vi "interface_configuration.vi"(8 "error in (no error)":errorcluster, 11 "config in":T1) -> (0 "error out":errorcluster, 3 "config out":T1)   [LabVIEW 2015, in "lv-builder-default.lvlib"]
uses:
  lv-builder-default.lvlib
  public/_controls/post_action_lvlib.ctl
  public/_controls/post_action_installer.ctl
  public/_controls/post_action_application.ctl
  public/_controls/post_action_zip.ctl
  public/_controls/configuration.ctl
  <vilib>/Utility/error.llb/Error Cluster From Error Code.vi
  <vilib>/ErrorRing/Error Ring.xnode
panel:
  in  "version":string caption="Version"
  in  "distribution_folder":path caption="Distribution Folder"
  in  "dependencies_folder":path caption="Dependencies Folder"
  in  "bin_folder":path caption="Bin Path"
  in  "application_post_action":T2 caption="Application Post Action"
  in  "cancel":bool
  in  "save":bool
  in  "installer_post_file":path caption="Installer Post File"
  in  "zip_move_directory":path caption="Archive Directory"
  in  "zip_post_action":T3 caption="Archive Post Action"
  in  "installer_post_action":T4 caption="Installer Post Action"
  in  "update_version_vi":path caption="Update Version VI"
  in  "lvlibp_move_directory":path caption="lvlibp Directory"
  in  "lvlib_move_directory":path caption="lvlib Directory"
  in  "lvlib_post_action":T5 caption="LVLIB Post Action"
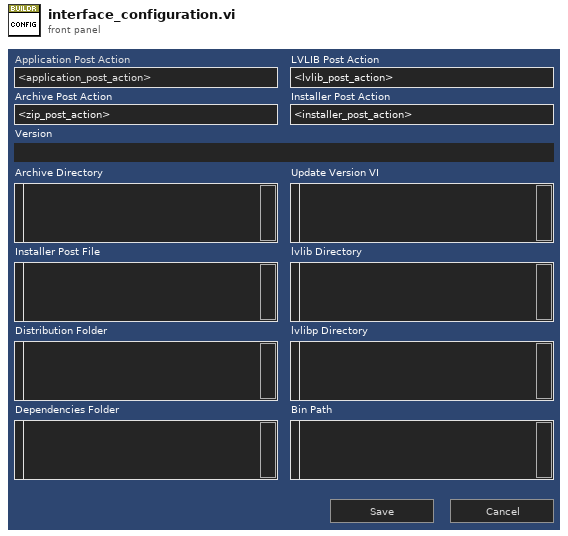
[diagram p1: front panel]
types:
  T1 = typedef "lv-builder-default.lvlib/configuration.ctl" = cluster{"project_file":string, "lvlibp_directory":string, "zip_directory":string, "lvlib_directory":string, "update_version_vi":string, "installer_post_file":string, "distribution_folder":string, "dependencies_folder":string, "version":string, "bin_folder":string, "lvlib_post_action":u16, "installer_post_action":u16, "application_post_action":u16, "zip_post_action":u16}
  T2 = typedef "lv-builder-default.lvlib/post_action_application.ctl" = enum16{"<application_post_action>", "nothing", "zip_application", "<null>"}
  T3 = typedef "lv-builder-default.lvlib/post_action_zip.ctl" = enum16{"<zip_post_action>", "nothing", "move", "extract", "<null>"}
  T4 = typedef "lv-builder-default.lvlib/post_action_installer.ctl" = enum16{"<installer_post_action>", "nothing", "create_installer", "zip_installer", "create_installer_file", "<null>"}
  T5 = typedef "lv-builder-default.lvlib/post_action_lvlib.ctl" = enum16{"<lvlib_post_action>", "nothing", "move", "install", "<null>"}
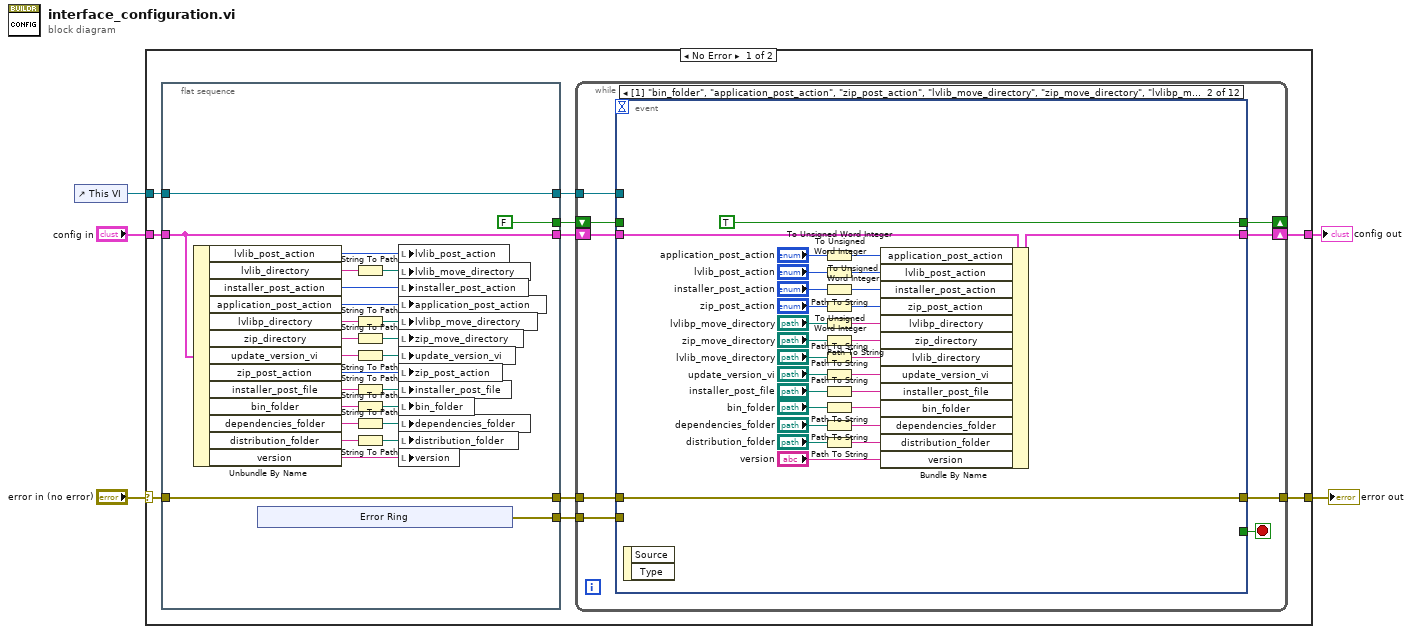
[diagram p0: block diagram]
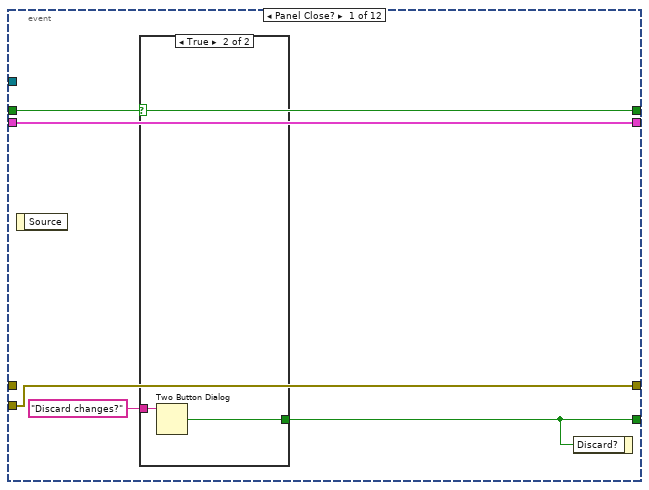
[diagram p2: hidden frame]
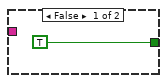
[diagram p3: hidden frame]
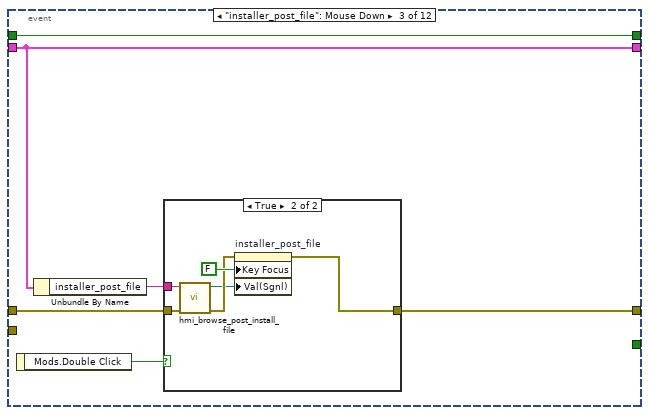
[diagram p4: hidden frame]
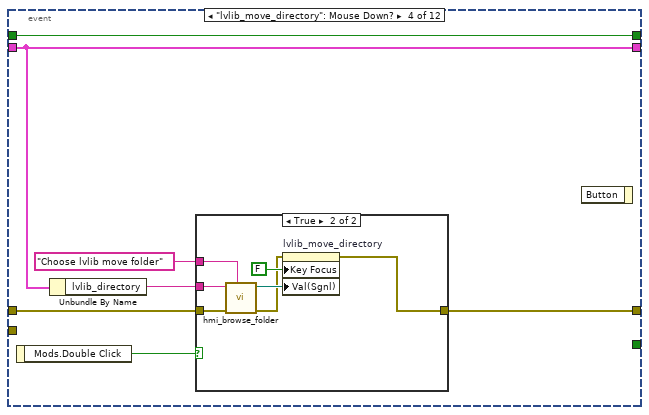
[diagram p6: hidden frame]
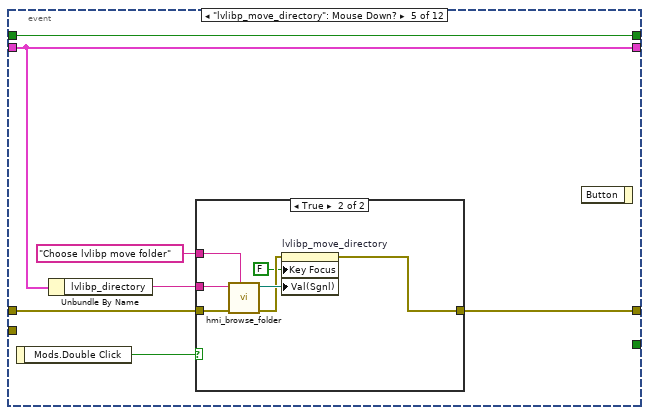
[diagram p8: hidden frame]
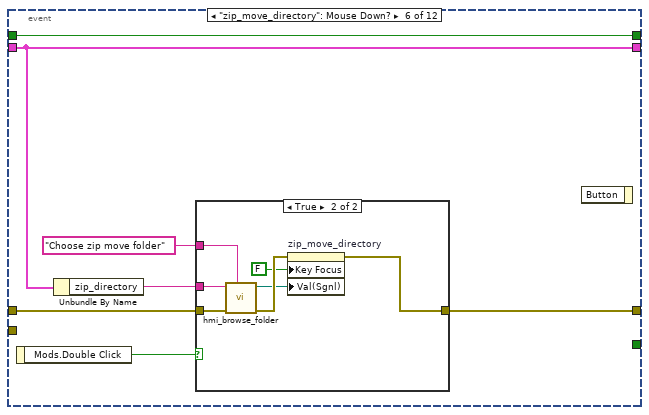
[diagram p10: hidden frame]
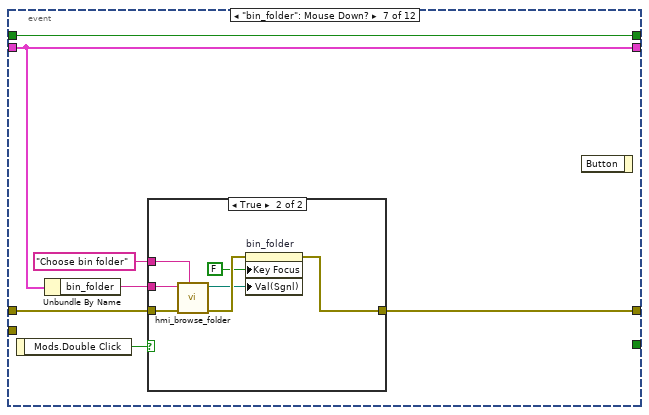
[diagram p12: hidden frame]
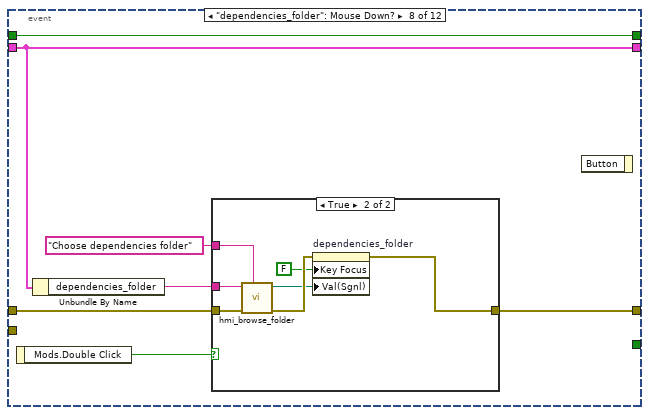
[diagram p14: hidden frame]
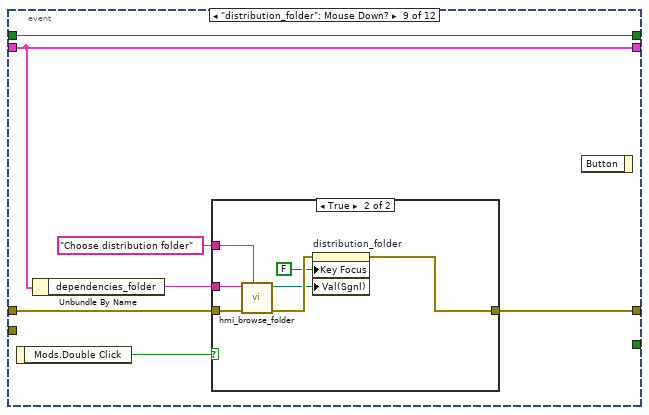
[diagram p16: hidden frame]
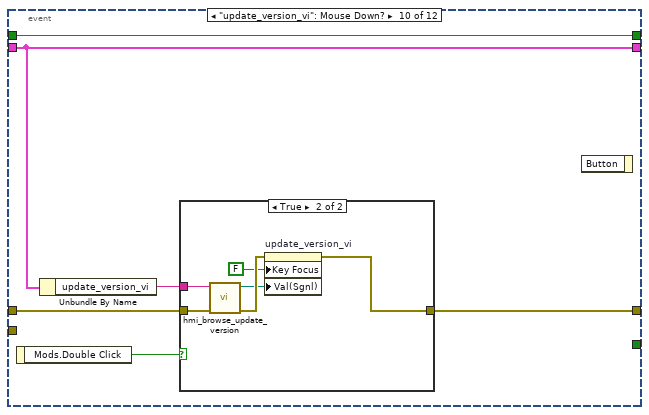
[diagram p18: hidden frame]
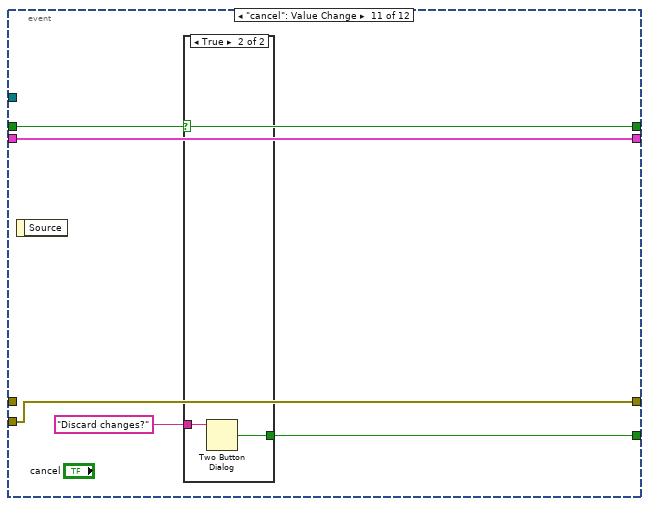
[diagram p20: hidden frame]
diagram:
  n1 = control-ref of="This VI"() -> (w3:refnum<vi>)
  n2 = case shown="No Error" "error in (no error)" {
    selector: "error in (no error)" -> [w15 w220]
    tunnel: [w9 w220] -> w4
    tunnel: w3 -> [w11 _]
    tunnel: [w8 _] -> w2
    tunnel: "config in" -> [w7 _]
    frame No Error {
      n3 = flat-sequence {
        tunnel: w15 -> [w24]
        tunnel: [w24] -> w14
        tunnel: [w25] -> w13
        tunnel: [w34] -> w12
        tunnel: w11 -> [w34]
        tunnel: [FALSE] -> w10
        tunnel: w7 -> [w25]
        tunnel: [w23] -> w6
        frame #0 {
          n4 = Unbundle By Name(w25) -> ("lvlib_post_action"=w35:u16, "lvlib_directory"=w40:string, "installer_post_action"=w36:u16, "application_post_action"=w37:u16, "lvlibp_directory"=w39:string, "zip_directory"=w38:string, "update_version_vi"=w33:string, "zip_post_action"=w32:u16, "installer_post_file"=w31:string, "bin_folder"=w22:string, "dependencies_folder"=w21:string, "distribution_folder"=w20:string, "version"=w16:string)
          n5 = xnode "Error Ring"() -> ("error out"=w23:errorcluster)
          n6 = String To Path(string=w40) -> (path=w30:path)
          n7 = String To Path(string=w39) -> (path=w29:path)
          n8 = String To Path(string=w38) -> (path=w28:path)
          n9 = String To Path(string=w33) -> (path=w27:path)
          n10 = String To Path(string=w31) -> (path=w26:path)
          n11 = String To Path(string=w22) -> (path=w19:path)
          n12 = String To Path(string=w21) -> (path=w18:path)
          n13 = String To Path(string=w20) -> (path=w17:path)
          n14 = local write "lvlib_post_action"(w35) -> ()
          n15 = local write "lvlib_move_directory"(w30) -> ()
          n16 = local write "installer_post_action"(w36) -> ()
          n17 = local write "application_post_action"(w37) -> ()
          n18 = local write "lvlibp_move_directory"(w29) -> ()
          n19 = local write "zip_move_directory"(w28) -> ()
          n20 = local write "update_version_vi"(w27) -> ()
          n21 = local write "zip_post_action"(w32) -> ()
          n22 = local write "installer_post_file"(w26) -> ()
          n23 = local write "bin_folder"(w19) -> ()
          n24 = local write "dependencies_folder"(w18) -> ()
          n25 = local write "distribution_folder"(w17) -> ()
          n26 = local write "version"(w16) -> ()
        }
      }
      n27 = while {
        tunnel: w14 -> [w47]
        shift-right: [w52] -> w8
        shift-left: w13 -> [w53]
        tunnel: w12 -> [w49]
        shift-right: [w50] -> _
        shift-left: w10 -> [w51]
        tunnel: [w48] -> w9
        tunnel: w6 -> [w46]
        stop <- w54 stop-if-true
        n28 = event shown="[1] \"bin_folder\", \"application_post_action\", \"zip_post_action\", \"lvlib_move_directory\", \"zip_move_directory\", \"lvlibp_move_directory\", \"update_version_vi\", \"installer_post_file\", \"installer_post_action\", \"dependencies_folder\", \"distribution_folder\", \"version\": Value Change" {
          selector: _ -> [_ _ _ _ _ _ _ _ _ _ _ _]
          dyn-events: _ -> [_ _ _ _ _ _ _ _ _ _ _ _]
          timeout: _ -> [_ _ _ _ _ _ _ _ _ _ _ _]
          tunnel: [w57 _ _ _ _ _ _ _ _ _ w212 TRUE ("Discard?")] -> w54
          tunnel: w49 -> [_ _ _ _ _ _ _ _ _ _ _ _]
          tunnel: w53 -> [w59 w91 w93 w105 w123 w138 w153 w168 w183 w198 w211 w218]
          tunnel: [w59 w89 w93 w105 w123 w138 w153 w168 w183 w198 w211 w218] -> w52
          tunnel: w51 -> [w56 _ w92 w106 w120 w135 w150 w165 w180 w195 w209 w219]
          tunnel: [w56 TRUE w92 w106 w120 w135 w150 w165 w180 w195 w209 w219] -> w50
          tunnel: [w55 w64 w94 w107 w121 w136 w151 w167 w182 w197 w208 w217] -> w48
          tunnel: w47 -> [_ w64 w95 w108 w122 w137 w152 w166 w181 w196 _ w217]
          tunnel: w46 -> [w55 _ _ _ _ _ _ _ _ _ w208 _]
          event Panel Close? {
            n29 = event-data() -> ()  [unwired: 1 in, 1 out]
            n30 = case shown="True" w56 {
              tunnel: [TRUE ("Discard?") w62] -> w57
              tunnel: "Discard changes?" ("dialog_text") -> [_ w61]
              frame False {
              }
              frame True {
                n31 = Two Button Dialog(message=w61) -> (T button?=w62:bool)  [unwired: 2 in]
              }
            }
            n32 = event-data("Discard?"=w57) -> ()  [unwired: 1 in, 1 out]
          }
          event "bin_folder", "lvlib_move_directory", "zip_move_directory", "lvlibp_move_directory", "update_version_vi", "installer_post_file", "dependencies_folder", "distribution_folder", "version": Value Change {
            n33 = event-data() -> ()  [unwired: 1 in, 2 out]
            n34 = To Unsigned Word Integer(number="application_post_action") -> (unsigned 16bit integer=w74:u16)
            n35 = To Unsigned Word Integer(number="lvlib_post_action") -> (unsigned 16bit integer=w73:u16)
            n36 = To Unsigned Word Integer(number="installer_post_action") -> (unsigned 16bit integer=w72:u16)
            n37 = To Unsigned Word Integer(number="zip_post_action") -> (unsigned 16bit integer=w71:u16)
            n38 = Path To String(path="lvlibp_move_directory") -> (string=w79:string)
            n39 = Path To String(path="zip_move_directory") -> (string=w78:string)
            n40 = Path To String(path="lvlib_move_directory") -> (string=w77:string)
            n41 = Path To String(path="update_version_vi") -> (string=w76:string)
            n42 = Path To String(path="installer_post_file") -> (string=w75:string)
            n43 = Path To String(path="bin_folder") -> (string=w65:string)
            n44 = Path To String(path="dependencies_folder") -> (string=w66:string)
            n45 = Path To String(path="distribution_folder") -> (string=w67:string)
            n46 = Bundle By Name(cluster=w91, "application_post_action"=w74, "lvlib_post_action"=w73, "installer_post_action"=w72, "zip_post_action"=w71, "lvlibp_directory"=w79, "zip_directory"=w78, "lvlib_directory"=w77, "update_version_vi"=w76, "installer_post_file"=w75, "bin_folder"=w65, "dependencies_folder"=w66, "distribution_folder"=w67, "version"="version") -> (w89:T1)
          }
          event "installer_post_file": Mouse Down {
            n47 = event-data() -> ("Mods.Double Click"=w97:bool)  [unwired: 1 in]
            n48 = Unbundle By Name(w93) -> ("installer_post_file"=w96:string)
            n49 = case shown="True" w97 {
              tunnel: w96 -> [_ w103]
              tunnel: w95 -> [w98 w102]
              tunnel: [w98 w99] -> w94
              frame False {
              }
              frame True {
                n50 = call "hmi_browse_post_install_file.vi"("error in (no error)"=w102, "post_installer_file"=w103) -> ("error out"=w101:errorcluster, "selected path"=w100:path)  [unwired: 8 in]
                n51 = property on="installer_post_file" class="Path"(error in=w101, "Key Focus"=FALSE, "Val(Sgnl)"=w100) -> (error out=w99:errorcluster)  [unwired: 1 in, 1 out]
              }
            }
          }
          event "lvlib_move_directory": Mouse Down? {
            n52 = event-data() -> ("Mods.Double Click"=w111:bool)  [unwired: 1 in]
            n53 = Unbundle By Name(w105) -> ("lvlib_directory"=w110:string)
            n54 = case shown="True" w111 {
              tunnel: w110 -> [_ w119]
              tunnel: "Choose lvlib move folder" ("description") -> [_ w118]
              tunnel: w108 -> [w112 w114]
              tunnel: [w112 w113] -> w107
              frame False {
              }
              frame True {
                n55 = call "hmi_browse_folder.vi"("description"=w118, "error in (no error)"=w114, "folder"=w119) -> ("error out"=w115:errorcluster, "selected path"=w116:path)  [unwired: 7 in]
                n56 = property on="lvlib_move_directory" class="Path"(error in=w115, "Key Focus"=FALSE, "Val(Sgnl)"=w116) -> (error out=w113:errorcluster)  [unwired: 1 in, 1 out]
              }
            }
            n57 = event-data() -> ()  [unwired: 2 in, 1 out]
          }
          event "lvlibp_move_directory": Mouse Down? {
            n58 = event-data() -> ("Mods.Double Click"=w126:bool)  [unwired: 1 in]
            n59 = Unbundle By Name(w123) -> ("lvlibp_directory"=w125:string)
            n60 = case shown="True" w126 {
              tunnel: w125 -> [_ w133]
              tunnel: "Choose lvlibp move folder" ("description") -> [_ w134]
              tunnel: w122 -> [w127 w132]
              tunnel: [w127 w129] -> w121
              frame False {
              }
              frame True {
                n61 = call "hmi_browse_folder.vi"("description"=w134, "error in (no error)"=w132, "folder"=w133) -> ("error out"=w130:errorcluster, "selected path"=w131:path)  [unwired: 7 in]
                n62 = property on="lvlibp_move_directory" class="Path"(error in=w130, "Key Focus"=FALSE, "Val(Sgnl)"=w131) -> (error out=w129:errorcluster)  [unwired: 1 in, 1 out]
              }
            }
            n63 = event-data() -> ()  [unwired: 2 in, 1 out]
          }
          event "zip_move_directory": Mouse Down? {
            n64 = event-data() -> ("Mods.Double Click"=w141:bool)  [unwired: 1 in]
            n65 = Unbundle By Name(w138) -> ("zip_directory"=w140:string)
            n66 = case shown="True" w141 {
              tunnel: w140 -> [_ w148]
              tunnel: "Choose zip move folder" ("description") -> [_ w149]
              tunnel: w137 -> [w142 w147]
              tunnel: [w142 w143] -> w136
              frame False {
              }
              frame True {
                n67 = call "hmi_browse_folder.vi"("description"=w149, "error in (no error)"=w147, "folder"=w148) -> ("error out"=w146:errorcluster, "selected path"=w145:path)  [unwired: 7 in]
                n68 = property on="zip_move_directory" class="Path"(error in=w146, "Key Focus"=FALSE, "Val(Sgnl)"=w145) -> (error out=w143:errorcluster)  [unwired: 1 in, 1 out]
              }
            }
            n69 = event-data() -> ()  [unwired: 2 in, 1 out]
          }
          event "bin_folder": Mouse Down? {
            n70 = event-data() -> ("Mods.Double Click"=w156:bool)  [unwired: 1 in]
            n71 = Unbundle By Name(w153) -> ("bin_folder"=w155:string)
            n72 = case shown="True" w156 {
              tunnel: w155 -> [_ w163]
              tunnel: "Choose bin folder" ("description") -> [_ w164]
              tunnel: w152 -> [w157 w160]
              tunnel: [w157 w158] -> w151
              frame False {
              }
              frame True {
                n73 = call "hmi_browse_folder.vi"("description"=w164, "error in (no error)"=w160, "folder"=w163) -> ("error out"=w162:errorcluster, "selected path"=w161:path)  [unwired: 7 in]
                n74 = property on="bin_folder" class="Path"(error in=w162, "Key Focus"=FALSE, "Val(Sgnl)"=w161) -> (error out=w158:errorcluster)  [unwired: 1 in, 1 out]
              }
            }
            n75 = event-data() -> ()  [unwired: 2 in, 1 out]
          }
          event "dependencies_folder": Mouse Down? {
            n76 = event-data() -> ("Mods.Double Click"=w171:bool)  [unwired: 1 in]
            n77 = Unbundle By Name(w168) -> ("dependencies_folder"=w170:string)
            n78 = case shown="True" w171 {
              tunnel: w170 -> [_ w178]
              tunnel: "Choose dependencies folder" ("description") -> [_ w179]
              tunnel: [w172 w173] -> w167
              tunnel: w166 -> [w172 w177]
              frame False {
              }
              frame True {
                n79 = call "hmi_browse_folder.vi"("description"=w179, "error in (no error)"=w177, "folder"=w178) -> ("error out"=w176:errorcluster, "selected path"=w175:path)  [unwired: 7 in]
                n80 = property on="dependencies_folder" class="Path"(error in=w176, "Key Focus"=FALSE, "Val(Sgnl)"=w175) -> (error out=w173:errorcluster)  [unwired: 1 in, 1 out]
              }
            }
            n81 = event-data() -> ()  [unwired: 2 in, 1 out]
          }
          event "distribution_folder": Mouse Down? {
            n82 = event-data() -> ("Mods.Double Click"=w186:bool)  [unwired: 1 in]
            n83 = Unbundle By Name(w183) -> ("dependencies_folder"=w185:string)
            n84 = case shown="True" w186 {
              tunnel: w185 -> [_ w193]
              tunnel: "Choose distribution folder" ("description") -> [_ w194]
              tunnel: [w187 w188] -> w182
              tunnel: w181 -> [w187 w192]
              frame False {
              }
              frame True {
                n85 = call "hmi_browse_folder.vi"("description"=w194, "error in (no error)"=w192, "folder"=w193) -> ("error out"=w191:errorcluster, "selected path"=w190:path)  [unwired: 7 in]
                n86 = property on="distribution_folder" class="Path"(error in=w191, "Key Focus"=FALSE, "Val(Sgnl)"=w190) -> (error out=w188:errorcluster)  [unwired: 1 in, 1 out]
              }
            }
            n87 = event-data() -> ()  [unwired: 2 in, 1 out]
          }
          event "update_version_vi": Mouse Down? {
            n88 = event-data() -> ("Mods.Double Click"=w200:bool)  [unwired: 1 in]
            n89 = Unbundle By Name(w198) -> ("update_version_vi"=w199:string)
            n90 = case shown="True" w200 {
              tunnel: w199 -> [_ w207]
              tunnel: [w201 w202] -> w197
              tunnel: w196 -> [w201 w206]
              frame False {
              }
              frame True {
                n91 = call "hmi_browse_update_version.vi"("error in (no error)"=w206, "update_version_vi"=w207) -> ("error out"=w205:errorcluster, "selected path"=w204:path)  [unwired: 8 in]
                n92 = property on="update_version_vi" class="Path"(error in=w205, "Key Focus"=FALSE, "Val(Sgnl)"=w204) -> (error out=w202:errorcluster)  [unwired: 1 in, 1 out]
              }
            }
            n93 = event-data() -> ()  [unwired: 2 in, 1 out]
          }
          event "cancel": Value Change {
            n94 = event-data() -> ()  [unwired: 1 in, 1 out]
            n95 = case shown="True" w209 {
              tunnel: [TRUE ("Discard?") w214] -> w212
              tunnel: "Discard changes?" ("dialog_text") -> [_ w215]
              frame False {
              }
              frame True {
                n96 = Two Button Dialog(message=w215) -> (T button?=w214:bool)  [unwired: 2 in]
              }
            }
          }
          event "save": Value Change {
            n97 = event-data() -> ()  [unwired: 1 in, 1 out]
          }
        }
      }
    }
    frame Error {
    }
  }
  "error out" <- w4
  "config out" <- w2
